vi "WAIT_BALL.vi"(10 "argv":string[](array[string]), 11 "args":u8) -> ()   [LabVIEW 2014]
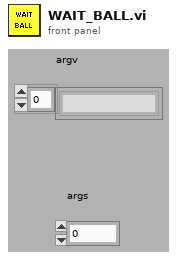
[diagram p1: front panel]
types:
  T1 = typedef "WPI_DigitalInputDevRef.ctl" = cluster{"DevStatus":errorcluster, "DIO Channel":T2, "Controller":T3}
  T2 = typedef "FPGA_DIOChannel.ctl" = enum8{"DIO 0", "DIO 1", "DIO 2", "DIO 3", "DIO 4", "DIO 5", "DIO 6", "DIO 7", "DIO 8", "DIO 9", "DIO MXP 0", "DIO MXP 1", "DIO MXP 2", "DIO MXP 3", "DIO MXP 4", "DIO MXP 5", "DIO MXP 6", "DIO MXP 7", "DIO MXP 8", "DIO MXP 9", "DIO MXP 10", "DIO MXP 11", "DIO MXP 12", "DIO MXP 13", "DIO MXP 14", "DIO MXP 15", "Invalid"}
  T3 = typedef "FPGA_TypedefDigitalModule.ctl" = enum16{"Controller 1"}
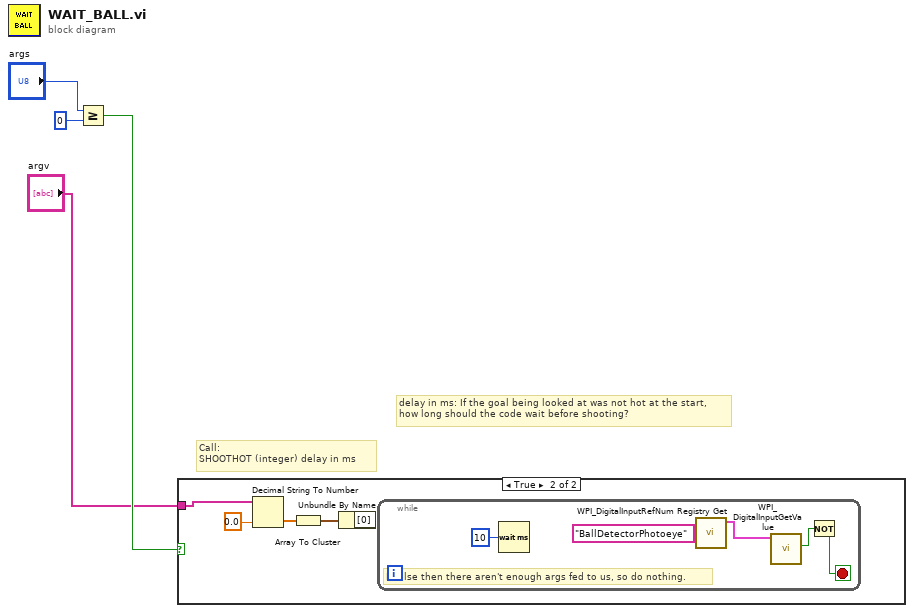
[diagram p0: block diagram]
diagram:
  # "delay in ms: If the goal being looked at was not hot at the start,\nhow long should the code wait before shooting?"
  # "Call:\nSHOOTHOT (integer) delay in ms"
  n1 = Greater Or Equal?(x="args", y=u8 0) -> (x >= y?=w4:bool)
  n2 = case shown="True" w4 {
    tunnel: "argv" -> [_ w5]
    frame False {
    }
    frame True {
      n3 = Decimal String To Number(string=w5, default (0L)=0.0 ("default (0 I32)")) -> (number=w7:dbl[])  [unwired: 2 out]
      n4 = Array To Cluster(array=w7) -> (cluster=w6:cluster{"[0]":dbl, "[1]":dbl})
      n5 = Unbundle By Name(w6) -> ()  [unwired: 1 out]
      n6 = while {
        stop <- w10 stop-if-true
        # "If false then there aren't enough args fed to us, so do nothing."
        n7 = Wait (ms)(milliseconds to wait=u32 10) -> ()  [unwired: 1 out]
        n8 = call <vilib>:"WPI_DigitalInputRefNum Registry Get.vi"("refnum name"="BallDetectorPhotoeye") -> ("DigitalInputDevRef"=w12:T1)  [unwired: 9 in, 1 out]
        n9 = call <vilib>:"WPI_DigitalInputGetValue.vi"("DigitalInputDevRef"=w12) -> ("Value"=w11:bool)  [unwired: 8 in, 2 out]
        n10 = Not(x=w11) -> (.not. x?=w10:bool)
      }
    }
  }
